vi "z_to_freq_damping.vi"(6 "Fs":dbl, 10 "Coefficients":dbl[](array[numeric]) format="%#_3g") -> (0 "Characteristics":T1 {"Frequency" format="%#_3p"; "Damping" min=0.0 max=1000.0 step=1.0 format="%#_3g"}, 2 "z location":cdb format="%#.3g", 3 "s location":cdb format="%#.3g")   [LabVIEW 2010]
uses:
  damping_freq.ctl
  <vilib>/analysis/polynomials.llb/Polynomial Roots (DBL).vi
  <vilib>/Analysis/NI_AALPro.lvlib
panel:
  # "Difference equation coefficients"
  # "Sampling frequency (1/sec)"
  # "Natural frequency (Hz)"
  # "Damping factor"
  # "Convert second order discrete time transfer function coefficients into natural frequency and damping factor representation.  This representation requires that real roots be identical."
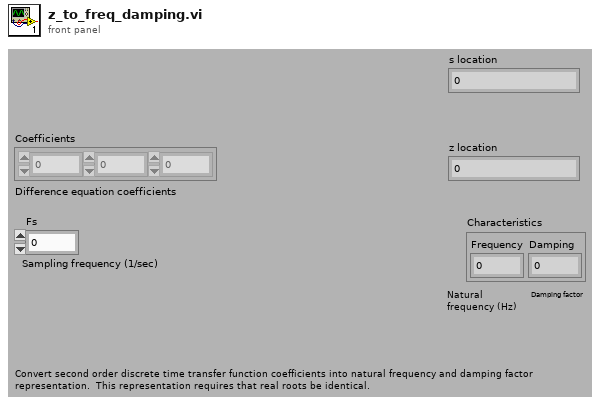
[diagram p1: front panel]
types:
  T1 = typedef "damping_freq.ctl" = cluster{"Frequency":dbl, "Damping":dbl}
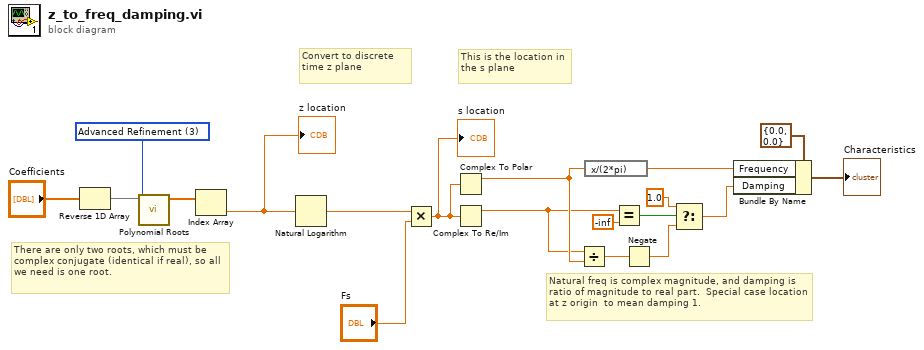
[diagram p0: block diagram]
diagram:
  w17 = u16 3 items=["General", "Simple Classification", "Refinement", "Advanced Refinement"] ("option")
  # "Natural freq is complex magnitude, and damping is ratio of magnitude to real part.  Special case location at z origin  to mean damping 1."
  # "There are only two roots, which must be complex conjugate (identical if real), so all we need is one root."
  # "Convert to discrete time z plane"
  # "This is the location in the s plane"
  n1 = Reverse 1D Array(array="Coefficients") -> (reversed array=w18:dbl[])
  n2 = call-poly <vilib>:"Polynomial Roots.vi"("option"=w17, "P(x)"=w18) -> ("Roots"=w16:cdb[])  [unwired: 9 out]
  n3 = Index Array(array=w16) -> (element=w8:cdb)  [unwired: 1 in]
  "z location" <- w8
  n4 = Natural Logarithm(1:w8) -> (0:w14:cdb)
  n5 = Multiply(x=w14, y="Fs") -> (x*y=w10:cdb)
  "s location" <- w10
  n6 = Complex To Polar(r * e^(i*theta)=w10) -> (r=w9:dbl)  [unwired: 1 out]
  n7 = Complex To Re/Im(x + iy=w10) -> (x=w6:dbl)  [unwired: 1 out]
  n8 = Divide(x=w6, y=w9) -> (x/y=w7:dbl)
  n9 = expression code="x/(2*pi)"(w9) -> (w13:dbl)
  n10 = Equal?(x=w6, y=-inf) -> (x = y?=w3:bool)
  n11 = Negate(x=w7) -> (-x=w1:dbl)
  n12 = Select(t=1.0 ("x"), s=w3, f=w1) -> (s? t:f=w4:dbl)
  n13 = Bundle By Name(cluster=T1 {"Frequency"=0.0, "Damping"=0.0} ("Characteristics"), "Frequency"=w13, "Damping"=w4) -> (→"Characteristics":T1)
